vi "TESTE.vi"() -> ()   [LabVIEW 2015]
uses:
  <vilib>/NXT/Subs/LVHSConnector.ctl
  <vilib>/NXT/LegoClasses/BrickReference/BrickReference.lvclass
  <vilib>/NXT/Block Support/NXT_ButtonSelector.ctl
  <vilib>/NXT/Block Support/NXT_InputPort.ctl
  <vilib>/NXT/Subs/MotorOutput.ctl
  <vilib>/NXT/Remote Library/Sound/NXT_SoundVolume.ctl
  <vilib>/NXT/Dual Mode Library/Display/drawText_Center.vi
  <vilib>/NXT/LegoClasses/EV3/LED Pattern.ctl
panel:
  in  "NXT/EV3 IN":T1
  out "NXT/EV3 OUT":T1
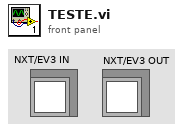
[diagram p1: front panel]
types:
  T1 = typedef "LVHSConnector.ctl" = refnum<class "BrickReference.lvclass">
  T2 = typedef "LED Pattern.ctl" = enum8{"None", "Green", "Red", "Orange", "Green Flash", "Red Flash", "Orange Flash", "Green Pulse", "Red Pulse", "Orange Pulse"}
  T3 = typedef "MotorOutput.ctl" = u8
  T4 = cluster{"PowerLeft":i32, "RotationLeft(Degrees)":i32, "PortLeft":T3}
  T5 = cluster{"PowerRight":i32, "RotationRight(Degrees)":i32, "PortRight":T3}
  T6 = typedef "NXT_ButtonSelector.ctl" = u16
  T7 = typedef "NXT_InputPort.ctl" = u32
  T8 = typedef "NXT_SoundVolume.ctl" = u8
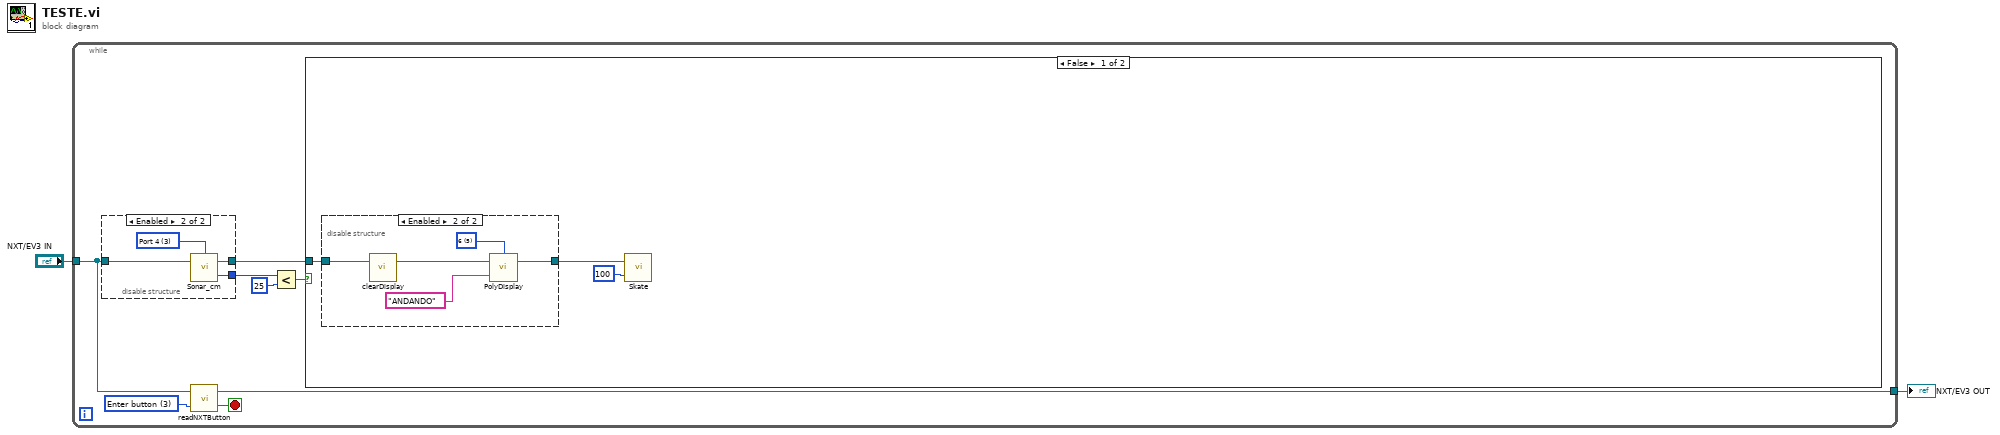
[diagram p0: block diagram]
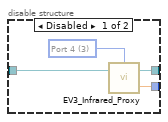
[diagram p2: hidden frame]
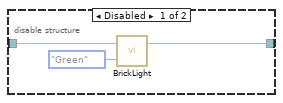
[diagram p3: hidden frame]
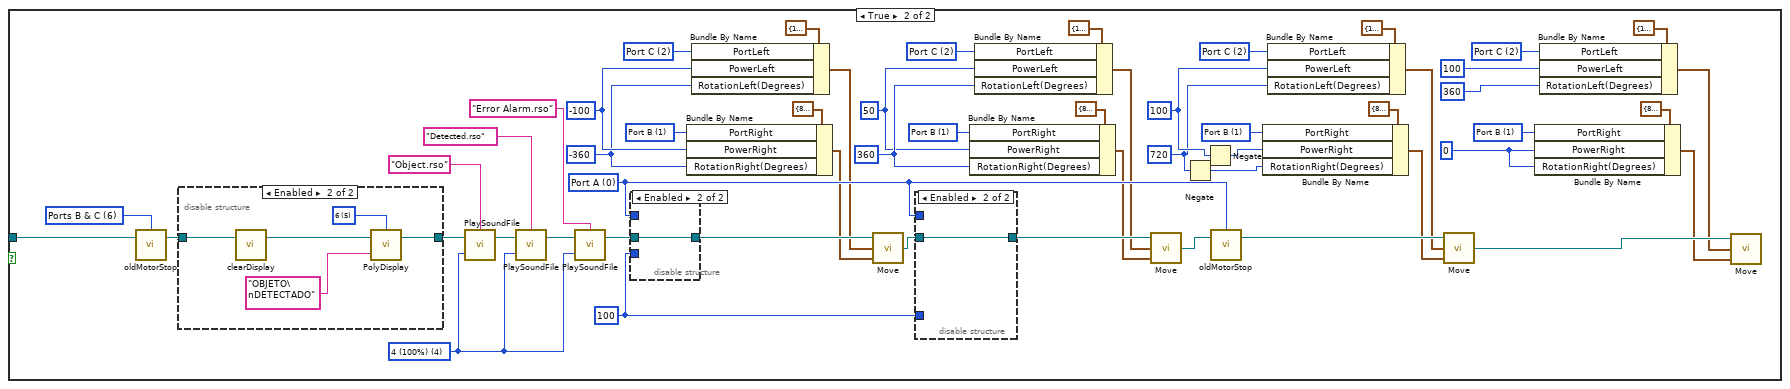
[diagram p4: hidden frame]
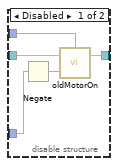
[diagram p5: hidden frame]
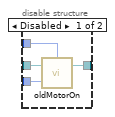
[diagram p6: hidden frame]
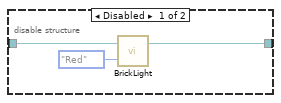
[diagram p7: hidden frame]
diagram:
  n1 = while {
    tunnel: "NXT/EV3 IN" -> [w5]
    tunnel: [w7] -> w2
    stop <- w10 stop-if-true
    w9 = T6 3 items=["Enter button"=3, "Left button"=2, "Right button"=1, "Up Button"=4, "Down Button"=5] ("Button (Enter button)")
    n2 = disable-structure shown="Enabled" {
      disable-tunnel: [w12 w18] -> w6
      disable-tunnel: w5 -> [w14 w17]
      disable-tunnel: [w11 w15] -> w4
      frame Disabled {
        w13 = T7 3 items=["Port 1", "Port 2", "Port 3", "Port 4"] ("Port (Port 1)")
        n3 = call <vilib>:"EV3_Infrared_Proxy.vi"("NXT/EV3"=w14, "Port (Port 1)"=w13) -> ("Scaled Value"=w11:sgl, "NXT/EV3"=w12:T1)  [unwired: 1 in]
      }
      frame Enabled {
        w16 = T7 3 items=["Port 1", "Port 2", "Port 3", "Port 4"] ("Port (Port 1)")
        n4 = call <vilib>:"Sonar_cm.vi"("NXT/EV3"=w17, "Port (Port 4)"=w16) -> ("Distance (cm)"=w15:i16, "NXT/EV3"=w18:T1)  [unwired: 1 in]
      }
    }
    n5 = call <vilib>:"readNXTButton.vi"("Button (Enter button)"=w9, "NXT/EV3"=w5) -> ("Yes/No"=w10:bool, "NXT/EV3"=w7:T1)  [unwired: 1 in]
    n6 = Less?(x=w4, y=i16 25) -> (x < y?=w8:bool)
    n7 = case shown="False" w8 {
      tunnel: w6 -> [w19 w83]
      frame False {
        n8 = disable-structure shown="Enabled" {
          disable-tunnel: [w23 w27] -> w20
          disable-tunnel: w19 -> [w22 w28]
          frame Disabled {
            n9 = call <vilib>:"BrickLight.vi"("Light Color"=LED_Pattern."Green", "NXT/EV3"=w22) -> ("NXT/EV3"=w23:T1)  [unwired: 2 in]
          }
          frame Enabled {
            w26 = i16 5 items=["1", "2", "3", "4", "5", "6", "7", "8", "9", "10", "11", "12"] ("Line")
            n10 = call <vilib>:"clearDisplay.vi"("NXT/EV3"=w28) -> ("NXT/EV3"=w29:T1)  [unwired: 3 in]
            n11 = call-poly <vilib>:"PolyDisplay.vi"("Text"="ANDANDO" ("Filename (*.ric)"), "NXT/EV3"=w29, "Line"=w26) -> ("NXT/EV3"=w27:T1)  [unwired: 1 in]
          }
        }
        n12 = call "Skate.vi"("Power"=100, "BrickReference in"=w20) -> ()  [unwired: 1 in, 1 out]
      }
      frame True {
        w33 = 0 ("PowerRight")
        w48 = T3 2 items=["Port A"=0, "Port B"=1, "Port C"=2, "Ports A & B"=4, "Ports A & C"=5, "Ports B & C"=6, "All Ports"=3] ("PortRight")
        w47 = T3 1 items=["Port A"=0, "Port B"=1, "Port C"=2, "Ports A & B"=4, "Ports A & C"=5, "Ports B & C"=6, "All Ports"=3] ("PortLeft")
        w39 = 100 ("PowerLeft")
        w37 = 720 ("RotationRight(Degrees)")
        w53 = T3 2 items=["Port A"=0, "Port B"=1, "Port C"=2, "Ports A & B"=4, "Ports A & C"=5, "Ports B & C"=6, "All Ports"=3] ("PortRight")
        w54 = T3 1 items=["Port A"=0, "Port B"=1, "Port C"=2, "Ports A & B"=4, "Ports A & C"=5, "Ports B & C"=6, "All Ports"=3] ("PortLeft")
        w30 = 50 ("PowerLeft")
        w43 = 360 ("RotationRight(Degrees)")
        w56 = T3 2 items=["Port A"=0, "Port B"=1, "Port C"=2, "Ports A & B"=4, "Ports A & C"=5, "Ports B & C"=6, "All Ports"=3] ("PortRight")
        w55 = T3 1 items=["Port A"=0, "Port B"=1, "Port C"=2, "Ports A & B"=4, "Ports A & C"=5, "Ports B & C"=6, "All Ports"=3] ("PortLeft")
        w65 = -100 ("PowerLeft")
        w64 = -360 ("RotationRight(Degrees)")
        w62 = T3 2 items=["Port A"=0, "Port B"=1, "Port C"=2, "Ports A & B"=4, "Ports A & C"=5, "Ports B & C"=6, "All Ports"=3] ("PortRight")
        w63 = T3 1 items=["Port A"=0, "Port B"=1, "Port C"=2, "Ports A & B"=4, "Ports A & C"=5, "Ports B & C"=6, "All Ports"=3] ("PortLeft")
        w59 = T3 0 items=["Port A"=0, "Port B"=1, "Port C"=2, "Ports A & B"=4, "Ports A & C"=5, "Ports B & C"=6, "All Ports"=3] ("Output Port (All Ports)")
        w70 = 100 ("Power (75)")
        w78 = T8 4 items=["0 (Mute)", "1 (25%)", "2 (50%)", "3 (75%)", "4 (100%)"] ("Volume (4)")
        w82 = T3 6 items=["Port A"=0, "Port B"=1, "Port C"=2, "Ports A & B"=4, "Ports A & C"=5, "Ports B & C"=6, "All Ports"=3] ("Output Port (All Ports)")
        n13 = call <vilib>:"oldMotorStop.vi"("NXT/EV3"=w83, "Output Port (All Ports)"=w82) -> ("NXT/EV3"=w75:T1)  [unwired: 2 in]
        n14 = disable-structure shown="Enabled" {
          disable-tunnel: [w96 w101] -> w74
          disable-tunnel: w75 -> [w95 w100]
          frame Disabled {
            n15 = call <vilib>:"BrickLight.vi"("Light Color"=LED_Pattern."Red", "NXT/EV3"=w95) -> ("NXT/EV3"=w96:T1)  [unwired: 2 in]
          }
          frame Enabled {
            w98 = i16 5 items=["1", "2", "3", "4", "5", "6", "7", "8", "9", "10", "11", "12"] ("Line")
            n16 = call <vilib>:"clearDisplay.vi"("NXT/EV3"=w100) -> ("NXT/EV3"=w102:T1)  [unwired: 3 in]
            n17 = call-poly <vilib>:"PolyDisplay.vi"("Text"="OBJETO\nDETECTADO" ("Filename (*.ric)"), "NXT/EV3"=w102, "Line"=w98) -> ("NXT/EV3"=w101:T1)  [unwired: 1 in]
          }
        }
        n18 = call <vilib>:"PlaySoundFile.vi"("Volume (4)"=w78, "NXT/EV3"=w74, "Filename (*.rso)"="Object.rso") -> ("NXT/EV3"=w79:T1)  [unwired: 1 in]
        n19 = call <vilib>:"PlaySoundFile.vi"("Volume (4)"=w78, "NXT/EV3"=w79, "Filename (*.rso)"="Detected.rso") -> ("NXT/EV3"=w77:T1)  [unwired: 1 in]
        n20 = call <vilib>:"PlaySoundFile.vi"("Volume (4)"=w78, "NXT/EV3"=w77, "Filename (*.rso)"="Error Alarm.rso") -> ("NXT/EV3"=w73:T1)  [unwired: 1 in]
        n21 = disable-structure shown="Enabled" {
          disable-tunnel: w59 -> [w93 _]
          disable-tunnel: w70 -> [w92 _]
          disable-tunnel: w73 -> [w91 w94]
          disable-tunnel: [w90 w94] -> w72
          frame Disabled {
            n22 = call <vilib>:"oldMotorOn.vi"("Power (75)"=w92, "NXT/EV3"=w91, "Output Port (All Ports)"=w93) -> ("NXT/EV3"=w90:T1)  [unwired: 1 in]
          }
          frame Enabled {
          }
        }
        n23 = Bundle By Name(cluster=T5 {"PowerRight"=80, "RotationRight(Degrees)"=360, "PortRight"=2} ("Right"), "PortRight"=w63, "PowerRight"=w65, "RotationRight(Degrees)"=w64) -> (w45:T5)
        n24 = Bundle By Name(cluster=T4 {"PowerLeft"=100, "RotationLeft(Degrees)"=360, "PortLeft"=1} ("Left"), "PortLeft"=w62, "PowerLeft"=w65, "RotationLeft(Degrees)"=w64) -> (w44:T4)
        n25 = call "Move.vi"("Right"=w45, "Left"=w44, "BrickReference in"=w72) -> ("BrickReference out"=w71:T1)
        n26 = disable-structure shown="Enabled" {
          disable-tunnel: w59 -> [w88 _]
          disable-tunnel: w71 -> [w87 w89]
          disable-tunnel: [w86 w89] -> w69
          disable-tunnel: w70 -> [w84 _]
          frame Disabled {
            n27 = Negate(x=w84) -> (-x=w85:i32)
            n28 = call <vilib>:"oldMotorOn.vi"("Power (75)"=w85, "NXT/EV3"=w87, "Output Port (All Ports)"=w88) -> ("NXT/EV3"=w86:T1)  [unwired: 1 in]
          }
          frame Enabled {
          }
        }
        n29 = Bundle By Name(cluster=T5 {"PowerRight"=80, "RotationRight(Degrees)"=360, "PortRight"=2} ("Right"), "PortRight"=w55, "PowerRight"=w30, "RotationRight(Degrees)"=w43) -> (w41:T5)
        n30 = Bundle By Name(cluster=T4 {"PowerLeft"=100, "RotationLeft(Degrees)"=360, "PortLeft"=1} ("Left"), "PortLeft"=w56, "PowerLeft"=w30, "RotationLeft(Degrees)"=w43) -> (w40:T4)
        n31 = call "Move.vi"("Right"=w41, "Left"=w40, "BrickReference in"=w69) -> ("BrickReference out"=w68:T1)
        n32 = Negate(x=w37) -> (-x=w36:i32)
        n33 = Negate(x=w39) -> (-x=w38:i32)
        n34 = call <vilib>:"oldMotorStop.vi"("NXT/EV3"=w68, "Output Port (All Ports)"=w59) -> ("NXT/EV3"=w66:T1)  [unwired: 2 in]
        n35 = Bundle By Name(cluster=T5 {"PowerRight"=80, "RotationRight(Degrees)"=360, "PortRight"=2} ("Right"), "PortRight"=w54, "PowerRight"=w38, "RotationRight(Degrees)"=w36) -> (w35:T5)
        n36 = Bundle By Name(cluster=T4 {"PowerLeft"=100, "RotationLeft(Degrees)"=360, "PortLeft"=1} ("Left"), "PortLeft"=w53, "PowerLeft"=w39, "RotationLeft(Degrees)"=w37) -> (w34:T4)
        n37 = call "Move.vi"("Right"=w35, "Left"=w34, "BrickReference in"=w66) -> ("BrickReference out"=w67:T1)
        n38 = Bundle By Name(cluster=T5 {"PowerRight"=80, "RotationRight(Degrees)"=360, "PortRight"=2} ("Right"), "PortRight"=w47, "PowerRight"=w33, "RotationRight(Degrees)"=w33) -> (w32:T5)
        n39 = Bundle By Name(cluster=T4 {"PowerLeft"=100, "RotationLeft(Degrees)"=360, "PortLeft"=1} ("Left"), "PortLeft"=w48, "PowerLeft"=100, "RotationLeft(Degrees)"=360 ("RotationRight(Degrees)")) -> (w31:T4)
        n40 = call "Move.vi"("Right"=w32, "Left"=w31, "BrickReference in"=w67) -> ()  [unwired: 1 out]
      }
    }
  }
  "NXT/EV3 OUT" <- w2
